vi "VCI_FindUsbDevice.vi"(8 "error in (no error)":errorcluster caption="错误输入（无错误）") -> (0 "error out":errorcluster caption="错误输出", 2 "VCI_BOARD_INFO1":T1, 3 "Total Devices":i32)   [LabVIEW 2018, in "ControlCan.lvlib"]
uses:
  ControlCan.lvlib
  VCI_BOARD_INFO1_1.ctl
  VCI_BOARD_INFO1.ctl
panel:
  in  "pInfo":T2
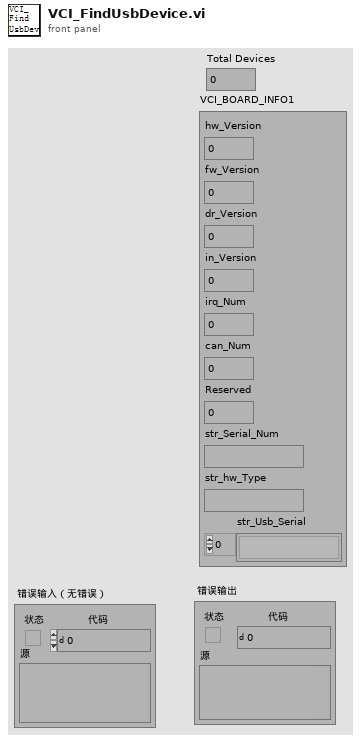
[diagram p1: front panel]
types:
  T1 = typedef "ControlCAN.lvlib/VCI_BOARD_INFO1.ctl" = cluster{"hw_Version":u16, "fw_Version":u16, "dr_Version":u16, "in_Version":u16, "irq_Num":u16, "can_Num":u8, "Reserved":u8, "str_Serial_Num":string, "str_hw_Type":string, "str_Usb_Serial":string[]}
  T2 = typedef "ControlCAN.lvlib/VCI_BOARD_INFO1_1.ctl" = cluster{"hw_Version":u16, "fw_Version":u16, "dr_Version":u16, "in_Version":u16, "irq_Num":u16, "can_Num":u8, "Reserved":u8, "str_Serial_Num 0":u8, "str_Serial_Num 1":u8, "str_Serial_Num 2":u8, "str_Serial_Num 3":u8, "str_Serial_Num 4":u8, "str_Serial_Num 5":u8, "str_Serial_Num 6":u8, "str_Serial_Num 7":u8, "str_hw_Type 0":u8, "str_hw_Type 1":u8, "str_hw_Type 2":u8, "str_hw_Type 3":u8, "str_hw_Type 4":u8, "str_hw_Type 5":u8, "str_hw_Type 6":u8, "str_hw_Type 7":u8, "str_hw_Type 8":u8, "str_hw_Type 9":u8, "str_hw_Type 10":u8, "str_hw_Type 11":u8, "str_hw_Type 12":u8, "str_hw_Type 13":u8, "str_hw_Type 14":u8, "str_hw_Type 15":u8, "str_Usb_Serial0 0":u8, "str_Usb_Serial0 1":u8, "str_Usb_Serial0 2":u8, "str_Usb_Serial0 3":u8, "str_Usb_Serial1 0":u8, "str_Usb_Serial1 1":u8, "str_Usb_Serial1 2":u8, "str_Usb_Serial1 3":u8, "str_Usb_Serial2 0":u8, "str_Usb_Serial2 1":u8, "str_Usb_Serial2 2":u8, "str_Usb_Serial2 3":u8, "str_Usb_Serial3 0":u8, "str_Usb_Serial3 1":u8, "str_Usb_Serial3 2":u8, "str_Usb_Serial3 3":u8}
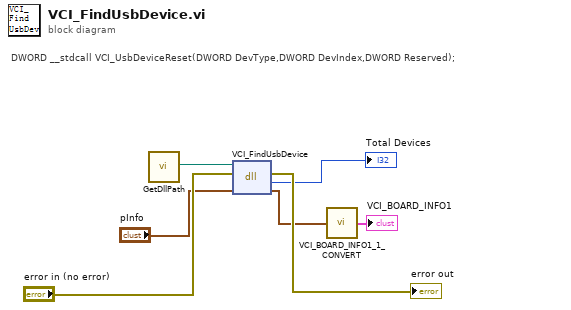
[diagram p0: block diagram]
diagram:
  # "DWORD __stdcall VCI_UsbDeviceReset(DWORD DevType,DWORD DevIndex,DWORD Reserved);"
  n1 = call "GetDllPath.vi"() -> ("DllPath"=w5:path)  [unwired: 1 in]
  n2 = dll-call lib="?" fn="VCI_FindUsbDevice"(path in=w5, error in="error in (no error)", "pInfo"="pInfo") -> (error out=→"error out":errorcluster, "Total Devices"=→"Total Devices":i32, "pInfo"=w2:T2)  [unwired: 1 in, 1 out]
  n3 = call "VCI_BOARD_INFO1_1_CONVERT.vi"("VCI_BOARD_INFO1_1"=w2) -> ("VCI_BOARD_INFO1"=→"VCI_BOARD_INFO1":T1)
